vi "send relative move to stage.vi"(8 "error in (no error)":errorcluster, 10 "move to send":dbl[unit], 11 "Cascade in":refnum<class "Cascade.lvclass">) -> (0 "error out":errorcluster, 3 "Cascade out":refnum<class "Cascade.lvclass">)   [LabVIEW 2012, in "Cascade.lvclass"]
uses:
  Cascade.lvclass
  <vilib>/Distrio/Murmex/GenericMessage/GenericMessage.lvclass
  Cascade.lvclass/Cascade.ctl
  <vilib>/Distrio/Murmex/Message/Message.lvclass
  <vilib>/Distrio/Murmex/Murmex/Murmex.lvclass
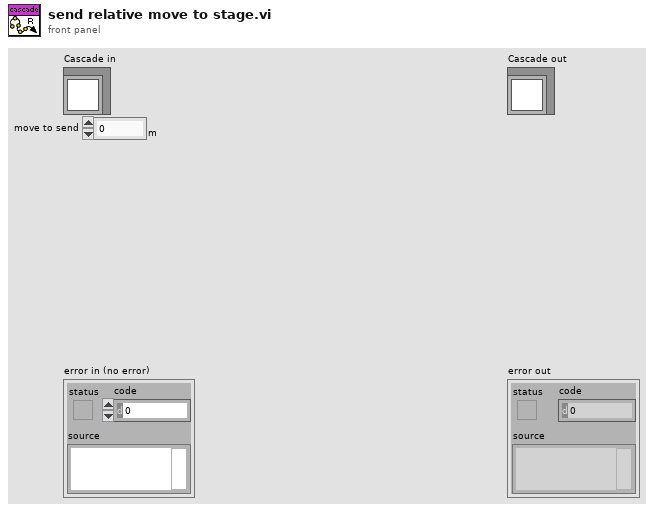
[diagram p1: front panel]
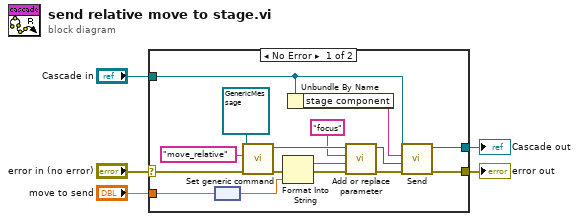
[diagram p0: block diagram]
diagram:
  n1 = case shown="No Error" "error in (no error)" {
    selector: "error in (no error)" -> [w12 w23]
    tunnel: [w11 w23] -> w4
    tunnel: [w8 w22] -> w2
    tunnel: "Cascade in" -> [w9 w22]
    tunnel: "move to send" -> [w7 _]
    frame No Error {
      n2 = node(w7) -> (w6:dbl)
      n3 = call <vilib>:"Set generic command.vi"("error in (no error)"=w12, "generic command"="move_relative" ("command string"), "GenericMessage in"=refnum<class "GenericMessage.lvclass"> refnum ("Murmex.lvlib:GenericMessage")) -> ("error out"=w18:errorcluster, "GenericMessage out"=w21:refnum<class "GenericMessage.lvclass">)  [unwired: 7 in]
      n4 = Format Into String(error in=w18, w6) -> (resulting string=w16:string, error out=w17:errorcluster)  [unwired: 2 in]
      n5 = Unbundle By Name(w9) -> ("stage component"=w10:string)
      n6 = call <vilib>:"Add or replace parameter.vi"("error in (no error)"=w17, "value"=w16, "name"="focus", "Message in"=w21) -> ("error out"=w19:errorcluster, "Message out"=w20:refnum<class "GenericMessage.lvclass">)  [unwired: 6 in]
      n7 = call <vilib>:"Send.vi"("error in (no error)"=w19, "Message"=w20, "recipient"=w10, "Murmex in"=w9) -> ("error out"=w11:errorcluster, "Murmex out"=w8:refnum<class "Cascade.lvclass">)  [unwired: 6 in]
    }
    frame Error {
    }
  }
  "error out" <- w4
  "Cascade out" <- w2
